vi "output.vi"(8 "error in":errorcluster, 10 "output data":T1, 11 "module in":refnum<class "user control module.lvclass">) -> (0 "error out":errorcluster, 2 "output allocation":T1, 3 "module out":refnum<class "user control module.lvclass">)   [LabVIEW 2013, in "user control module.lvclass"]
doc: "Provides an interface for writing data to a module at runtime. While this interface performs no operations, a child should provide an override which may write to any open sessions, references, or interfaces."
uses:
  user control module.lvclass
  <vilib>/NI/Tag Bus/table/data table.ctl
  <vilib>/NI/Tag Bus/table/data table.lvlib
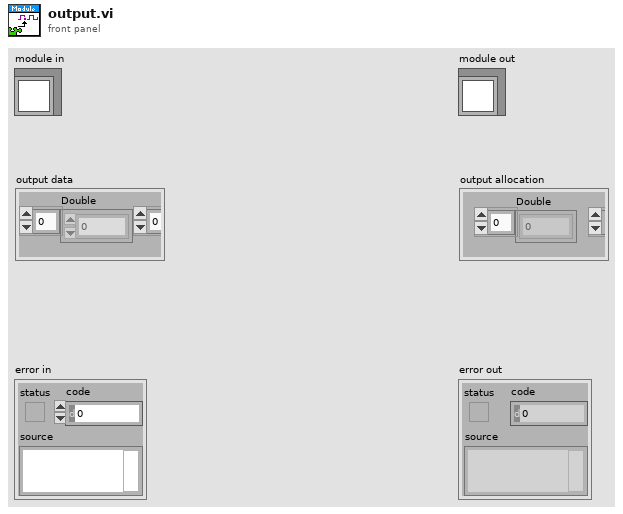
[diagram p1: front panel]
types:
  T1 = typedef "tag bus.lvlib/data table.lvlib/data table.ctl" = cluster{"Double":dbl[], "Single":sgl[], "I64":i64[], "I32":i32[], "I16":i16[], "I8":i8[], "U64":u64[], "U32":u32[], "U16":u16[], "U8":u8[], "Boolean":bool[], "String":string[], "Array of Double":cluster{"DBL Array":dbl[]}[], "Array of Single":cluster{"SGL Array":sgl[]}[], "Array of I64":cluster{"I64 Array":i64[]}[], "Array of I32":cluster{"I32 Array":i32[]}[], "Array of I16":cluster{"I16 Array":i16[]}[], "Array of I8":cluster{"I8 Array":i8[]}[], "Array of U64":cluster{"U64 Array":u64[]}[], "Array of U32":cluster{"U32 Array":u32[]}[], "Array of U16":cluster{"U16 Array":u16[]}[], "Array of U8":cluster{"U8 Array":u8[]}[], "Array of Boolean":cluster{"Boolean Array":bool[]}[], "Array of String":cluster{"String Array":string[]}[]}
  T2 = typedef "user control module configuration.lvclass/output data indices.ctl" = cluster{"Single.placeholder":i32}
  T3 = typedef "user control module.lvclass/output user data.ctl" = cluster{"fmwk_placeholder":sgl}
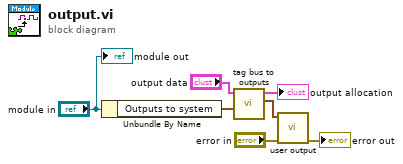
[diagram p0: block diagram]
diagram:
  n1 = Unbundle By Name("module in") -> ("Outputs to system"=w5:T2)
  n2 = call "tag bus to outputs.vi"("indices"=w5, "tag bus in"="output data") -> ("data cluster"=w3:T3, "tag bus out"=→"output allocation":T1)  [unwired: 8 in]
  n3 = call "user output.vi"("error in"="error in", "Outputs to system"=w3) -> ("error out"=→"error out":errorcluster)  [unwired: 9 in]
  "module out" <- "module in"
